vi "GFITS_SetCompression.vi"(10 "cmd in":string, 11 "Database RefNum out":T1) -> ()   [LabVIEW 2016]
uses:
  DBSHAND/private/vis/DatabaseHand_RefNum.ctl
  DBSHAND/private/vis/DatabaseHand_Element_Set(string).vi
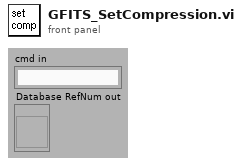
[diagram p1: front panel]
types:
  T1 = typedef "DatabaseHand_RefNum.ctl" = refnum<vi>
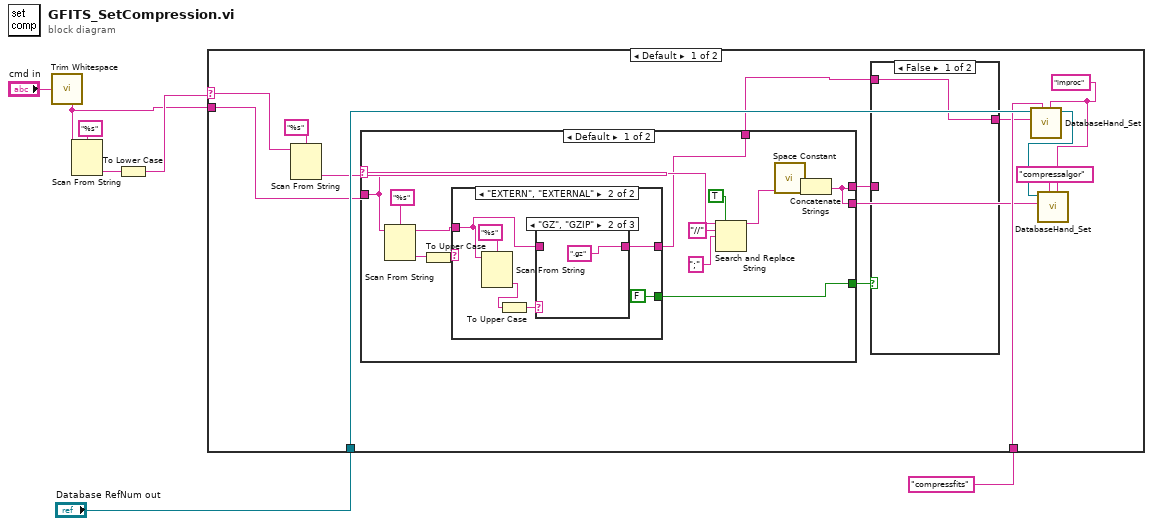
[diagram p0: block diagram]
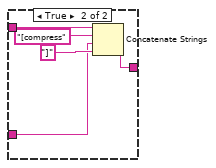
[diagram p2: hidden frame]
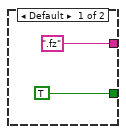
[diagram p3: hidden frame]
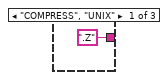
[diagram p4: hidden frame]
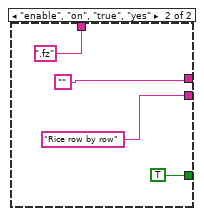
[diagram p6: hidden frame]
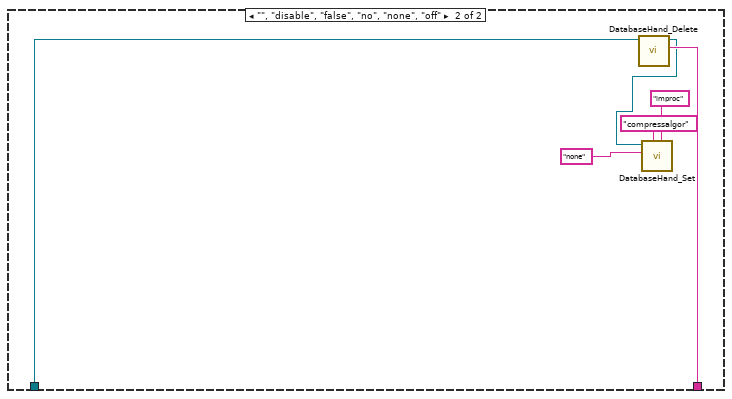
[diagram p7: hidden frame]
diagram:
  n1 = call <vilib>:"Trim Whitespace.vi"("string"="cmd in") -> ("trimmed string"=w4:string)  [unwired: 1 in]
  n2 = Scan From String(format string="%s" ("Format String"), input string=w4) -> (output 1=w6:string)  [unwired: 2 in, 4 out]
  n3 = To Lower Case(string=w6) -> (all lower case string=w5:string)
  n4 = case shown="Default" w5 {
    selector: w5 -> [w18 _]
    tunnel: w4 -> [w15 _]
    tunnel: "Database RefNum out" -> [w21 w61]
    tunnel: "compressfits" ("name") -> [w20 w60]
    frame Default {
      w13 = "improc" ("group")
      n5 = Scan From String(format string="%s", input string=w18) -> (output 1=w16:string)  [unwired: 2 in, 4 out]
      n6 = case shown="Default" w16 {
        tunnel: [w30 ""] -> w10
        tunnel: w15 -> [w35 _]
        tunnel: [w31 ".fz"] -> w14
        tunnel: [w30 "Rice row by row" ("name")] -> w9
        tunnel: [w29 TRUE ("replace all? (F)")] -> w8
        frame Default {
          n7 = Scan From String(format string="%s", input string=w35) -> (remaining string=w28:string, output 1=w33:string)  [unwired: 2 in, 3 out]
          n8 = To Upper Case(1:w33) -> (0:w32:string)
          n9 = case shown="\"EXTERN\", \"EXTERNAL\"" w32 {
            tunnel: [".fz" w44] -> w31
            tunnel: [TRUE ("replace all? (F)") FALSE ("replace all? (F)")] -> w29
            tunnel: w28 -> [_ w43]
            frame Default {
            }
            frame "EXTERN", "EXTERNAL" {
              n10 = Scan From String(format string="%s", input string=w43) -> (output 1=w47:string)  [unwired: 2 in, 4 out]
              n11 = To Upper Case(1:w47) -> (0:w46:string)
              n12 = case shown="\"GZ\", \"GZIP\"" w46 {
                tunnel: [".Z" ".gz" w51] -> w44
                tunnel: w43 -> [_ _ w51]
                frame "COMPRESS", "UNIX" {
                }
                frame "GZ", "GZIP" {
                }
                frame Default {
                }
              }
            }
          }
          n13 = Search and Replace String(replace all?=TRUE ("replace all? (F)"), input string=w35, search string="//", replace string=";" ("replace string (\"\")")) -> (result string=w39:string)  [unwired: 1 in, 6 out]
          n14 = call <vilib>:"Space Constant.vi"() -> ("String"=w40:string)
          n15 = Concatenate Strings(w40, w39) -> (w30:string)
        }
        frame "enable", "on", "true", "yes" {
        }
      }
      n16 = case shown="False" w8 {
        tunnel: [w22 w25] -> w19
        tunnel: w14 -> [w22 w24]
        tunnel: w10 -> [_ w23]
        frame False {
        }
        frame True {
          n17 = Concatenate Strings(w24, "[compress" ("string"), w23, "]" ("string")) -> (w25:string)
        }
      }
      n18 = call-poly "DatabaseHand_Set.vi"("group"=w13, "name"=w20, "value"=w19, "Database RefNum in"=w21) -> ("Database RefNum out"=w12:T1)  [unwired: 4 in, 3 out]
      n19 = call-poly "DatabaseHand_Set.vi"("group"=w13, "name"="compressalgor", "value"=w9, "Database RefNum in"=w12) -> ()  [unwired: 4 in, 4 out]
    }
    frame "", "disable", "false", "no", "none", "off" {
      n20 = call "DatabaseHand_Delete.vi"("name"=w60, "Database RefNum in"=w61) -> ("Database RefNum out"=w58:T1)  [unwired: 1 in, 8 out]
      n21 = call-poly "DatabaseHand_Set.vi"("group"="improc", "name"="compressalgor", "value"="none", "Database RefNum in"=w58) -> ()  [unwired: 4 in, 4 out]
    }
  }
